vi "Set XNET Properties.vi"(8 "error in (no error)":errorcluster, 10 "J1939 XNET Settings":T1={"XNET Database"="", "XNET Cluster"="", "CAN Port"="", "Baud rate [Bd]"=0, "J1939 Network Address"=0, "Name"=0, "Termination"=0, "Incoming Rate"=100, "Outcoming Rate"=100} {"Termination" items=["Off", "On"]}, 11 "Custom Device ref in":refnum<k24>) -> (0 "error out":errorcluster, 3 "Custom Device ref out":refnum<k24>)   [LabVIEW 2013, in "J1939 System Definition API Support.lvlib"]
uses:
  J1939 System Definition API Support.lvlib
  NationalInstruments.VeriStand.SystemDefinitionAPI
  Shared/Types/XNET Settings.ctl
  Shared/SubVIs/Constants.vi
  <vilib>/NI Veristand/Custom Device API/Set Item Property (Variant).vi
  <vilib>/NI Veristand/Custom Device API/Custom Device API.lvlib
  Shared/J1939 Addon Shared.lvlib
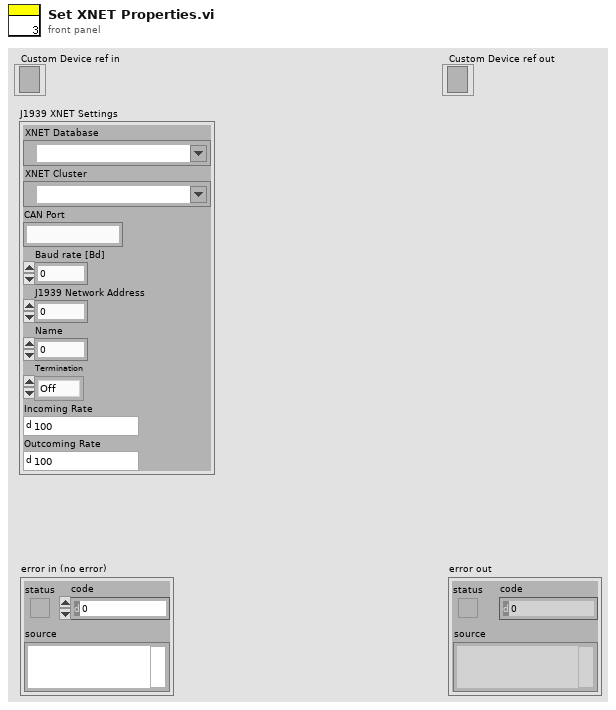
[diagram p1: front panel]
types:
  T1 = typedef "J1939 Addon Shared.lvlib/XNET Settings.ctl" = cluster{"XNET Database":refnum<k21>, "XNET Cluster":refnum<k21>, "CAN Port":string, "Baud rate [Bd]":u32, "J1939 Network Address":u8, "Name":u64, "Termination":u32, "Incoming Rate":u32, "Outcoming Rate":u32}
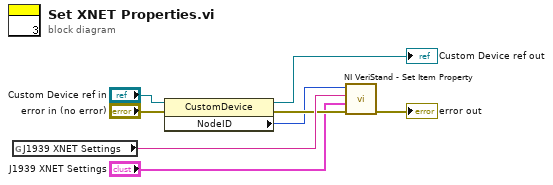
[diagram p0: block diagram]
diagram:
  n1 = global read "Constants.vi" "J1939 XNET Settings"() -> (w5:string)
  n2 = property class="CustomDevice"(reference="Custom Device ref in", error in="error in (no error)") -> (reference out=→"Custom Device ref out":refnum<k24>, error out=w4:errorcluster, "NodeID"=w3:u64)
  n3 = call-poly <vilib>:"NI VeriStand - Set Item Property.vi"("error in (no error)"=w4, "Value"="J1939 XNET Settings", "Property Name"=w5, "Item Ref in"=w3) -> ("error out"=→"error out":errorcluster)  [unwired: 5 in, 2 out]
